vi "Sort Teams by Number.vi"(11 "Team Info":T1) -> (3 "Array":T2[](array[typedef]))   [LabVIEW 2013]
uses:
  Team Data.ctl
  Team Data Array.ctl
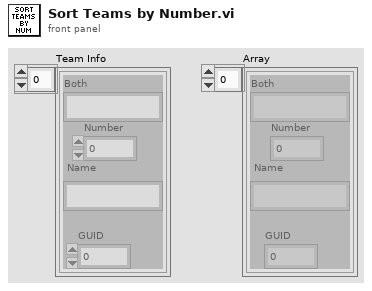
[diagram p1: front panel]
types:
  T1 = typedef "Team Data Array.ctl" = T2[]
  T2 = typedef "Team Data.ctl" = cluster{"Both":string, "Name":string, "GUID":u16, "Number":u16}
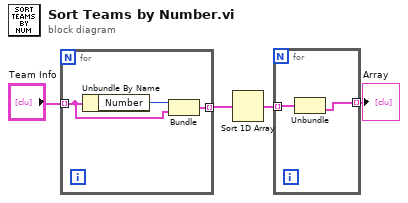
[diagram p0: block diagram]
diagram:
  n1 = for {
    tunnel: "Team Info" -> [w7] mode=indexing
    tunnel: [w5] -> w2 mode=indexing
    n2 = Unbundle By Name(w7) -> ("Number"=w6:u16)
    n3 = Bundle("Number"=w6, "Team Dataasd"=w7) -> (w5:cluster{"Number":u16, "Team Dataasd":T2})  [unwired: 1 in]
  }
  n4 = Sort 1D Array(array=w2) -> (sorted array=w3:cluster{"Number":u16, "Team Dataasd":T2}[])
  n5 = for {
    tunnel: w3 -> [w9] mode=indexing
    tunnel: [w8] -> w4 mode=indexing
    n6 = Unbundle(w9) -> ("Team Dataasd"=w8:T2)  [unwired: 1 out]
  }
  "Array" <- w4
